vi "eDIDS-24XX-Diesel-Host.vi"() -> ()   [LabVIEW 2015]
uses:
  <vilib>/addons/Software Calibration Management/XControls/SubHost List.xctl
  <vilib>/addons/Software Calibration Management/XControls/SubHost.xctl
panel:
  out "EngineStatus":u8
  in  "EngineSpeed_MaxNC":sgl
  out "5VPSU_CriticalFault":bool
  out "12VPSU_CriticalFault":bool
  out "BattV_CriticalFault":bool
  out "Inj1Duration":sgl[](array[numeric])
  in  "EngineSpeed_MaxCrit":sgl
  out "_Engine Speed":sgl
  out "EngineSpeedFPGA1":sgl(knob) scale=0.0..5000.0 scale format="%#_6p"
  in  "ESTOP":bool caption="Push to Stop"
  out "_5VPresent":bool caption="5V"
  out "_12VPresent":bool caption="12V"
  out "Critical Fault":bool
  out "Non-Critical Fault":bool
  out "_BattVPresent":bool caption="Battery"
  out "SyncFPGA1":bool caption="Sync"
  out "ReceivingPrimaryFPGA1":bool caption="Rcvg Primary"
  in  "_Main Tab":enum32{"Runtime", "Setup"}(tab)
  out "Software Version":string caption="Version:"
  in  "Control":T1(xcontrol)
  in  "System":T1(xcontrol)
  in  "Hardware":T1(xcontrol)
  out "_Engine Control Version":string caption="Version:"
  in  "Engine":T1(xcontrol)
  in  "Engine Time Reset":bool
  out "Time Since Start":sgl caption="[sec]" format="%05.0f"
  out "Engine Time":sgl caption="[hr]" format="%0#5_4f"
  in  "SyncEnable":bool caption="Sync Enable"
  out "MAF":sgl caption="[kg/hr]"
  in  "MEP_ManE":bool
  in  "MEP_Man":sgl(slide) caption="[bar]" scale=0.0..25.0
  out "OilT":sgl caption="[C]"
  out "MAT":sgl caption="[C]"
  out "OilP":sgl caption="[kPa]"
  out "ECT":sgl caption="[C]"
  out "UEGO1Lambda":sgl caption="[]"
  out "_Cyl1 Main Inj. Dur.":sgl caption="Cyl1 Main Inj. Dur."
  out "Fuel_Des":sgl caption="[mg/cyc]"
  out "EGRMass":sgl caption="[mg/cyc]"
  out "EGRMass_Des":sgl caption="[mg/cyc]"
  out "RailP":sgl caption="[bar]"
  out "RailP_Des":sgl caption="[bar]"
  out "MEP_Des":sgl caption="[bar]"
  out "MAP":sgl caption="[kPa]"
  out "MAP_Des":sgl caption="[kPa]"
  out "_EngineStatus":enum32{"A", "B", "C"}(ring)
  in  "_SubHost Tab":T2(tab)
  in  "NI 9862 (XNET CAN)":T3(xcontrol)
  in  "NI 9754-2 (ESTTL)":T3(xcontrol)
  in  "NI 9754-1 (ESTTL)":T3(xcontrol)
  in  "VR / Hall":T3(xcontrol)
  in  "NI 9411-1 (Digital Input)":T3(xcontrol)
  in  "NI 9758-2 (PFI/LS)":T3(xcontrol)
  in  "NI 9751-4 (DI Driver)":T3(xcontrol)
  in  "NI 9751-3 (DI Driver)":T3(xcontrol)
  in  "NI 9751-2 (DI Driver)":T3(xcontrol)
  in  "NI 9220-1 (AI)":T3(xcontrol)
  in  "NI 9757 (O2)":T3(xcontrol)
  in  "NI 9411-3 (Digital Input)":T3(xcontrol)
  in  "NI 9411-2 (Digital Input)":T3(xcontrol)
  in  "NI 9759 (Throttle)":T3(xcontrol)
  in  "NI 9758-1 (PFI/LS)":T3(xcontrol)
  in  "NI 9751-1 (DI Driver)":T3(xcontrol)
  in  "EPTx":T3(xcontrol)
  in  "EGR Actuation":T3(xcontrol)
  in  "Direct Injectors":T3(xcontrol)
  in  "Boost Actuation":T3(xcontrol)
  in  "Variable Valve Actuation":T3(xcontrol)
  in  "Engine Specs":T3(xcontrol)
  in  "Sensors":T3(xcontrol)
  in  "High Pressure Common Rail":T3(xcontrol)
  in  "Faults":T3(xcontrol) caption="0"
  in  "EGR Control":T3(xcontrol) caption="5"
  in  "Cranking":T3(xcontrol) caption="0"
  in  "Wastegate Control":T3(xcontrol) caption="6"
  in  "VGT Control":T3(xcontrol) caption="6"
  in  "Intake Air Desired":T3(xcontrol) caption="5"
  in  "DI Control":T3(xcontrol) caption="2"
  in  "Fuel Command":T3(xcontrol) caption="1"
  in  "Load Command":T3(xcontrol) caption="0"
  in  "Intake Air Measured":T3(xcontrol) caption="1"
  in  "EGR Flow":T3(xcontrol) caption="5"
  in  "VVT/VVA Control":T3(xcontrol) caption="9"
  in  "Rail Pressure Control":T3(xcontrol) caption="4"
  in  "Execution Info":T3(xcontrol)
  in  "Calscope and Trends":T3(xcontrol)
  # "[msec]"
  # "RPM"
  # "Version:"
  # "Version:"
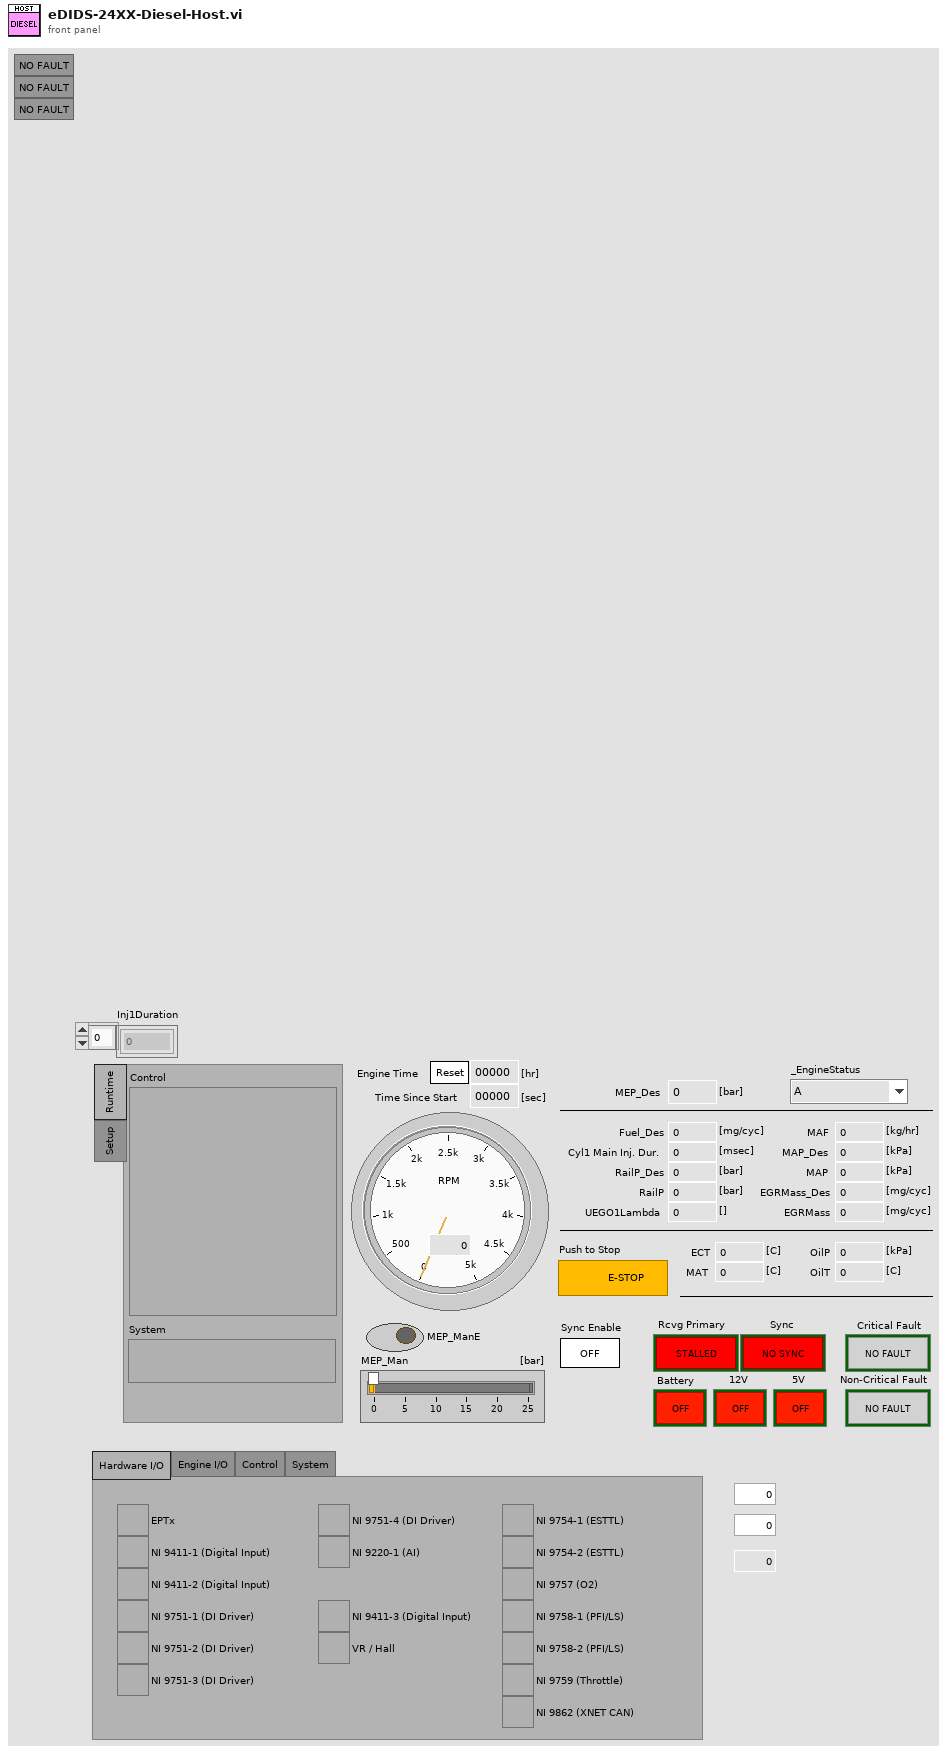
[diagram p1: front panel]
types:
  T1 = cluster{"States":enum32{"Invalid", "Standard", "Closed", "Hidden", "Minimized", "Maximized"}[], "VI Names":string[], "VI Refnums":refnum<vi>[], "Sub-Host Group":string, "Scrollbar":bool, "Listbox":refnum<vi>}
  T2 = enum32{"Hardware I/O", "Engine I/O", "Control", "System"}
  T3 = cluster{"Name":string, "Host VI":path, "Pairing File":path, "Display Name":string}
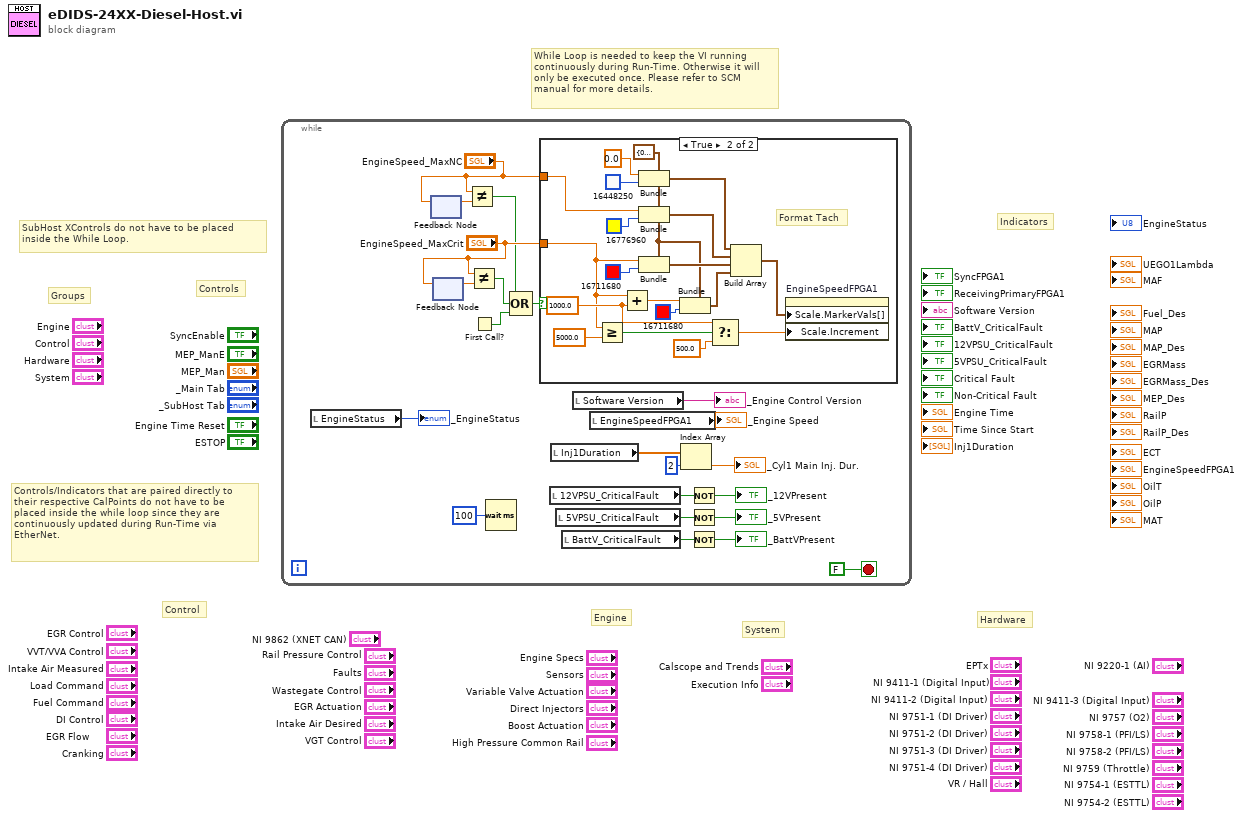
[diagram p0: block diagram]
diagram:
  # "Controls"
  # "Indicators"
  # "Groups"
  # "System"
  # "Hardware"
  # "Engine"
  # "Control"
  # "Controls/Indicators that are paired directly to their respective CalPoints do not have to be placed inside the while loop since they are continuously updated during Run-Time via EtherNet."
  # "While Loop is needed to keep the VI running\ncontinuously during Run-Time. Otherwise it will only be executed once. Please refer to SCM manual for more details."
  # "SubHost XControls do not have to be placed inside the While Loop."
  n1 = while {
    stop <- FALSE stop-if-true
    n2 = local read "EngineStatus"() -> (→"_EngineStatus":u8)
    n3 = feedback #1() -> (w7:sgl)  [unwired: 1 in]
    n4 = feedback-in #1("EngineSpeed_MaxNC") -> ()
    n5 = feedback #2() -> (w18:sgl)  [unwired: 1 in]
    n6 = feedback-in #2("EngineSpeed_MaxCrit") -> ()
    n7 = Not Equal?(x="EngineSpeed_MaxNC", y=w7) -> (x != y?=w4:bool)
    n8 = Not Equal?(x="EngineSpeed_MaxCrit", y=w18) -> (x != y?=w3:bool)
    n9 = First Call?() -> (First Call?: T/F=w5:bool)
    n10 = Wait (ms)(milliseconds to wait=u32 100) -> ()  [unwired: 1 out]
    n11 = Compound Arithmetic op=OR(w4, w3, w5) -> (w6:bool)
    n12 = case shown="True" w6 {
      tunnel: "EngineSpeed_MaxCrit" -> [_ w30]
      tunnel: "EngineSpeed_MaxNC" -> [_ w24]
      frame False {
      }
      frame True {
        w31 = sgl 1000.0 ("y")
        w27 = cluster{dbl, u32} {0.0, 0}
        # "Format Tach"
        n13 = Greater Or Equal?(x=w30, y=sgl 5000.0) -> (x >= y?=w33:bool)
        n14 = Add(x=w30, y=w31) -> (x+y=w35:sgl)
        n15 = Bundle(cluster=w27, sgl 0.0, u32 16448250) -> (w26:cluster{dbl, u32})
        n16 = Bundle(cluster=w27, w24, u32 16776960) -> (w25:cluster{dbl, u32})
        n17 = Bundle(cluster=w27, w30, u32 16711680) -> (w41:cluster{dbl, u32})
        n18 = Bundle(cluster=w27, w35, u32 16711680) -> (w38:cluster{dbl, u32})
        n19 = Select(t=w31, s=w33, f=sgl 500.0 ("Scale.Range:Increment")) -> (s? t:f=w28:sgl)
        n20 = Build Array(w26, w25, w41, w38) -> (w29:cluster{dbl, u32}[])
        n21 = property on="EngineSpeedFPGA1" class="Knob (strict)"("Scale.MarkerVals[]"=w29, "Scale.Increment"=w28) -> ()  [unwired: 2 in, 2 out]
      }
    }
    n22 = local read "12VPSU_CriticalFault"() -> (w11:bool)
    n23 = local read "Inj1Duration"() -> (w15:sgl[])
    n24 = local read "5VPSU_CriticalFault"() -> (w12:bool)
    n25 = local read "BattV_CriticalFault"() -> (w13:bool)
    n26 = local read "Software Version"() -> (→"_Engine Control Version":string)
    n27 = local read "EngineSpeedFPGA1"() -> (→"_Engine Speed":sgl)
    n28 = Index Array(array=w15, index=2) -> (element=→"_Cyl1 Main Inj. Dur.":sgl)
    n29 = Not(x=w11) -> (.not. x?=→"_12VPresent":bool)
    n30 = Not(x=w12) -> (.not. x?=→"_5VPresent":bool)
    n31 = Not(x=w13) -> (.not. x?=→"_BattVPresent":bool)
  }
